vi "Get Cal Coefficients.vi"(11 "Path":path) -> (0 "Error Out":errorcluster, 2 "PrevCalDate":i32, 3 "Cal Coefficients":dbl[][](array[numeric]))   [LabVIEW 2013]
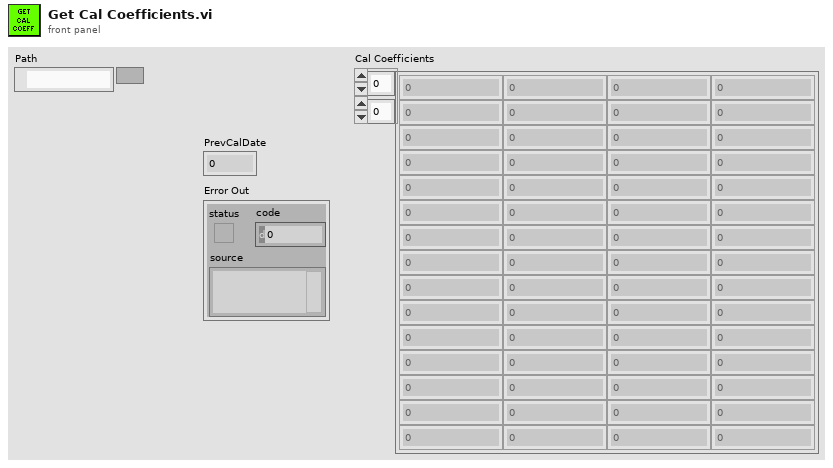
[diagram p1: front panel]
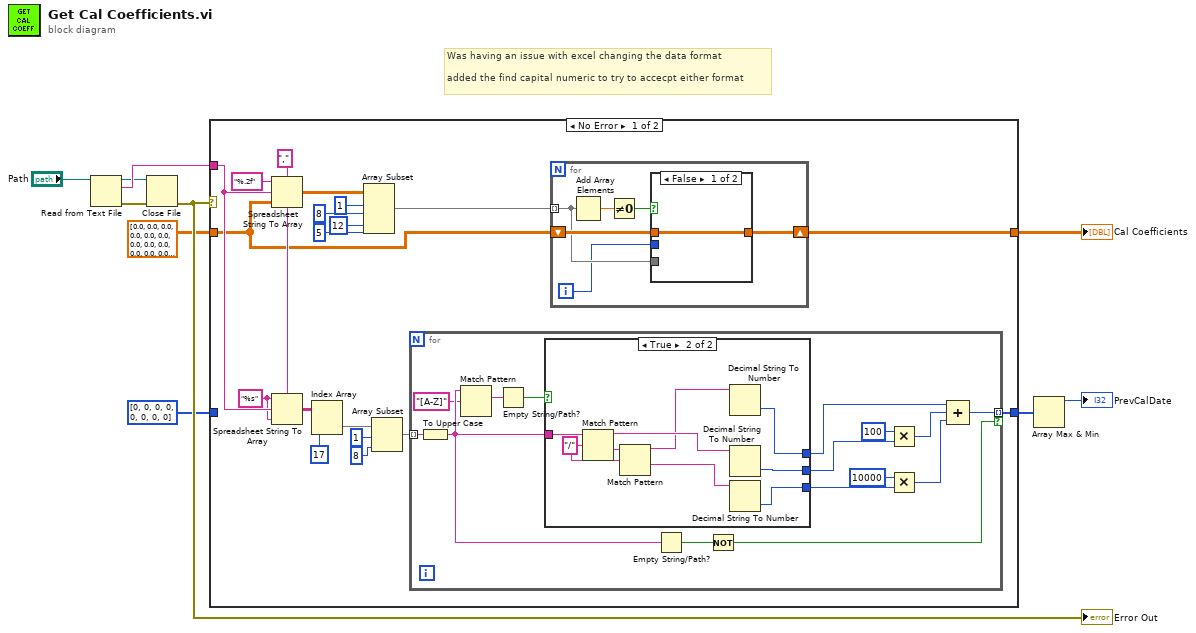
[diagram p0: block diagram]
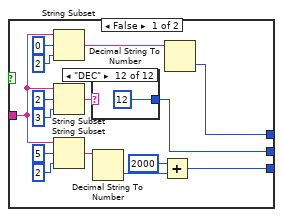
[diagram p2: hidden frame]
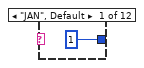
[diagram p3: hidden frame]
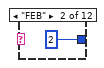
[diagram p4: hidden frame]
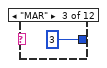
[diagram p5: hidden frame]
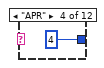
[diagram p6: hidden frame]
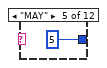
[diagram p7: hidden frame]
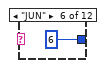
[diagram p8: hidden frame]
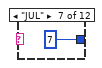
[diagram p9: hidden frame]
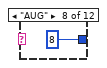
[diagram p10: hidden frame]
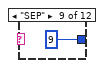
[diagram p11: hidden frame]
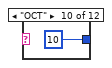
[diagram p12: hidden frame]
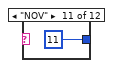
[diagram p13: hidden frame]
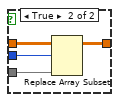
[diagram p14: hidden frame]
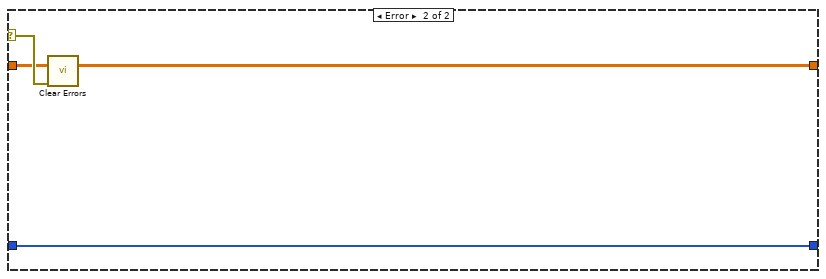
[diagram p15: hidden frame]
diagram:
  # "Was having an issue with excel changing the data format\n\nadded the find capital numeric to try to accecpt either format"
  n1 = Read from Text File(file (use dialog)="Path") -> (refnum out=w8:refnum<file>, text=w9:string, error out=w7:errorcluster)  [unwired: 3 in, 1 out]
  n2 = Close File(refnum=w8, error in=w7) -> (error out=w10:errorcluster)  [unwired: 1 out]
  "Error Out" <- w10
  n3 = case shown="No Error" w10 {
    selector: w10 -> [_ w94]
    tunnel: w9 -> [w23 _]
    tunnel: [w12 w92] -> w4
    tunnel: [w13 w93] -> w3
    tunnel: i32[] [0, 0, 0, 0, 0, 0, 0, 0] -> [_ w93]
    tunnel: dbl[][] [[0.0, 0.0, 0.0, 0.0, 0.0], [0.0, 0.0, 0.0, 0.0, 0.0], [0.0, 0.0, 0.0, 0.0, 0.0], [0.0, 0.0, 0.0, 0.0, 0.0], [0.0, 0.0, 0.0, 0.0, 0.0], [0.0, 0.0, 0.0, 0.0, 0.0], [0.0, 0.0, 0.0, 0.0, 0.0], [0.0, 0.0, 0.0, 0.0, 0.0]] -> [w11 w92]
    frame No Error {
      w20 = "%s" ("format string")
      w22 = "," ("delimiter (Tab)")
      n4 = Spreadsheet String To Array(delimiter (Tab)=w22, format string="%.2f", spreadsheet string=w23, array type (2D Dbl)=w11) -> (array=w27:dbl[][])
      n5 = Spreadsheet String To Array(delimiter (Tab)=w22, format string=w20, spreadsheet string=w23, array type (2D Dbl)=w20) -> (array=w16:string[][])
      n6 = Index Array(array=w16, index (col)=17 ("disabled index (col)")) -> (element=w14:string[])  [unwired: 1 in]
      n7 = Array Subset(array=w27, index (row)=1 ("index"), length (row)=8 ("length"), index (col)=12 ("index"), length (col)=5 ("length")) -> (w24:dbl[][])
      n8 = Array Subset(array=w14, index=1, length=8) -> (w17:string[])
      n9 = for {
        tunnel: w17 -> [w42] mode=indexing
        tunnel: [w30] -> w13 mode=indexing if=w43
        n10 = To Upper Case(1:w42) -> (0:w41:string)
        n11 = Match Pattern(string=w41, regular expression="[A-Z]") -> (match substring=w39:string)  [unwired: 1 in, 3 out]
        n12 = Empty String/Path?(string/path=w39) -> (empty?=w38:bool)
        n13 = case shown="True" w38 {
          tunnel: [w59 w80] -> w34
          tunnel: [w58 w79] -> w33
          tunnel: [w57 w78] -> w35
          tunnel: w41 -> [w56 w77]
          frame False {
            n14 = String Subset(string=w56, offset (0)=0, length (rest)=2 ("length (rest)")) -> (substring=w45:string)
            n15 = String Subset(string=w56, offset (0)=2, length (rest)=3 ("length (rest)")) -> (substring=w50:string)
            n16 = String Subset(string=w56, offset (0)=5, length (rest)=2 ("length (rest)")) -> (substring=w49:string)
            n17 = case shown="\"DEC\"" w50 {
              tunnel: [1 ("month") 2 ("month") 3 ("month") 4 ("month") 5 ("month") 6 ("month") 7 ("month") 8 ("month") 9 ("month") 10 ("month") 11 ("month") 12 ("month")] -> w59
              frame "JAN", Default {
              }
              frame "FEB" {
              }
              frame "MAR" {
              }
              frame "APR" {
              }
              frame "MAY" {
              }
              frame "JUN" {
              }
              frame "JUL" {
              }
              frame "AUG" {
              }
              frame "SEP" {
              }
              frame "OCT" {
              }
              frame "NOV" {
              }
              frame "DEC" {
              }
            }
            n18 = Decimal String To Number(string=w49) -> (number=w48:i32)  [unwired: 2 in, 1 out]
            n19 = Add(x=2000 ("year"), y=w48) -> (x+y=w58:i32)
            n20 = Decimal String To Number(string=w45) -> (number=w57:i32)  [unwired: 2 in, 1 out]
          }
          frame True {
            w75 = "/" ("regular expression")
            n21 = Match Pattern(string=w77, regular expression=w75) -> (before substring=w74:string, after substring=w76:string)  [unwired: 1 in, 2 out]
            n22 = Match Pattern(string=w76, regular expression=w75) -> (before substring=w73:string, after substring=w72:string)  [unwired: 1 in, 2 out]
            n23 = Decimal String To Number(string=w73) -> (number=w78:i32)  [unwired: 2 in, 1 out]
            n24 = Decimal String To Number(string=w74) -> (number=w80:i32)  [unwired: 2 in, 1 out]
            n25 = Decimal String To Number(string=w72) -> (number=w79:i32)  [unwired: 2 in, 1 out]
          }
        }
        n26 = Empty String/Path?(string/path=w41) -> (empty?=w44:bool)
        n27 = Not(x=w44) -> (.not. x?=w43:bool)
        n28 = Multiply(x=100, y=w34) -> (x*y=w36:i32)
        n29 = Multiply(x=10000, y=w33) -> (x*y=w37:i32)
        n30 = Compound Arithmetic op=ADD(w35, w36, w37) -> (w30:i32)
      }
      n31 = for {
        tunnel: w24 -> [w83] mode=indexing
        shift-right: [w81] -> w12
        shift-left: w11 -> [w84]
        i -> [w82]
        n32 = Add Array Elements(numeric array=w83) -> (sum=w86:dbl)
        n33 = Not Equal To 0?(x=w86) -> (x != 0?=w85:bool)
        n34 = case shown="False" w85 {
          tunnel: w84 -> [w87 w91]
          tunnel: w83 -> [_ w90]
          tunnel: w82 -> [_ w89]
          tunnel: [w87 w88] -> w81
          frame False {
          }
          frame True {
            n35 = Replace Array Subset(array=w91, new element=w90, index (row)=w89) -> (w88:dbl[][])  [unwired: 1 in]
          }
        }
      }
    }
    frame Error {
      n36 = call <vilib>:"Clear Errors.vi"("error in (no error)"=w94) -> ()  [unwired: 6 in, 1 out]
    }
  }
  "Cal Coefficients" <- w4
  n37 = Array Max & Min(array=w3) -> (max value=→"PrevCalDate":i32)  [unwired: 3 out]
